vi "Substract(U64).vi"(1 "Enable(T)":bool=TRUE, 2 "In":u64, 4 "n":u64=1) -> (6 "Out":u64=1)   [LabVIEW 2013]
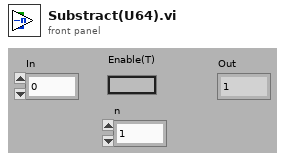
[diagram p1: front panel]
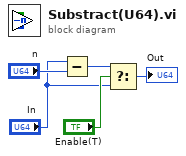
[diagram p0: block diagram]
diagram:
  n1 = Subtract(x="In", y="n") -> (x-y=w1:u64)
  n2 = Select(t=w1, s="Enable(T)", f="In") -> (s? t:f=→"Out":u64)
